vi "Calc.vi"(8 "error in (no error)":errorcluster, 10 "ArrayOfWVFMs":waveform(dbl)[](array[waveform]), 11 "RMS in":refnum<class "RMS.lvclass">) -> (0 "error out":errorcluster, 2 "Results":string[](array[string]), 3 "RMS out":refnum<class "RMS.lvclass">)   [LabVIEW 2015, in "RMSLib.lvlib" / "RMS.lvclass"]
uses:
  RMS.lvclass
  <vilib>/Analysis/5stat.llb/RMS (DBL).vi
  <vilib>/Analysis/NI_AALPro.lvlib
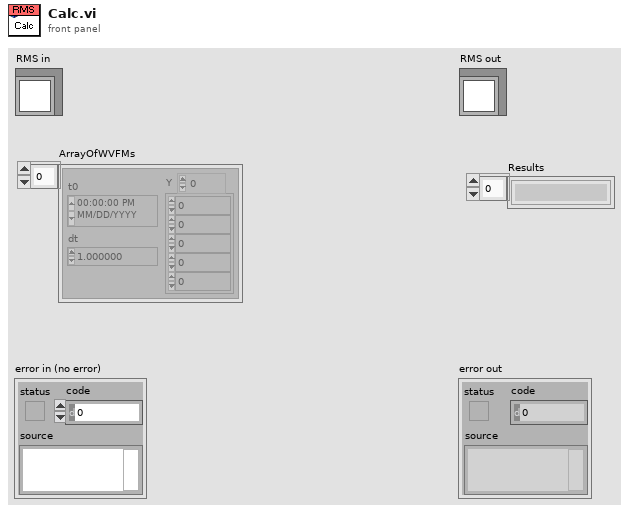
[diagram p1: front panel]
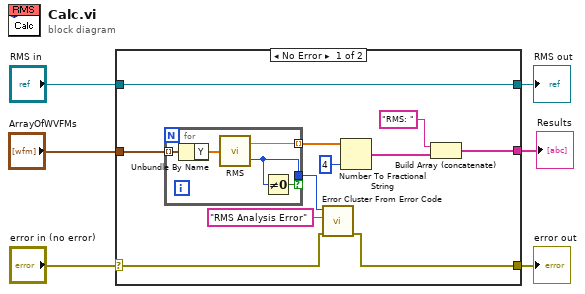
[diagram p0: block diagram]
diagram:
  n1 = case shown="No Error" "error in (no error)" {
    selector: "error in (no error)" -> [w14 w23]
    tunnel: "RMS in" -> [w17 w24]
    tunnel: [w17 w24] -> w4
    tunnel: [w13 w23] -> w3
    tunnel: "ArrayOfWVFMs" -> [w10 _]
    tunnel: [w8 _] -> w1
    frame No Error {
      n2 = for {
        tunnel: w10 -> [w19] mode=indexing
        tunnel: [w20] -> w16 if=w21
        tunnel: [w22] -> w12 mode=indexing
        n3 = Unbundle By Name(w19) -> ("Y"=w18:dbl[])
        n4 = call-poly <vilib>:"RMS.vi"("X"=w18) -> ("rms value"=w22:dbl, "error"=w20:i32)
        n5 = Not Equal To 0?(x=w20) -> (x != 0?=w21:bool)
      }
      n6 = call <vilib>:"Error Cluster From Error Code.vi"("error in (no error)"=w14, "error message (\"\")"="RMS Analysis Error" ("error message (\"\")"), "error code (0)"=w16) -> ("error out"=w13:errorcluster)  [unwired: 6 in]
      n7 = Number To Fractional String(number=w12, precision (6)=i16 4) -> (F-format string=w9:string[])  [unwired: 2 in]
      n8 = Build Array (concatenate)("RMS: ", w9) -> (w8:string[])
    }
    frame Error {
    }
  }
  "error out" <- w3
  "RMS out" <- w4
  "Results" <- w1
